vi "PQbinaryTuples.vi"(8 "error in (no error)":errorcluster, 10 "res":u64) -> (0 "error out":errorcluster, 1 "PQbinaryTuples":i64, 2 "res out":u64)   [LabVIEW 2019, in "libpqlv64.lvlib"]
doc: "Returns 1 if the PGresult contains binary data and 0 if it contains text data.\nThis function is deprecated (except for its use in connection with COPY), because it is possible for a single PGresult to contain text data in some columns and binary data in others. PQfformat is preferred. PQbinaryTuples returns 1 only if all columns of the result are binary (format 1)."
uses:
  libpqlv64.lvlib
  libpq.dll
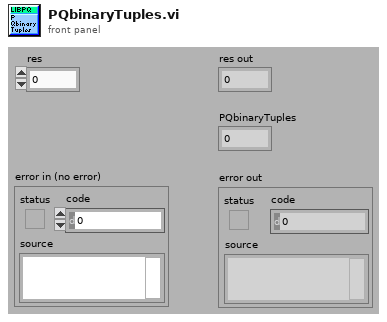
[diagram p1: front panel]
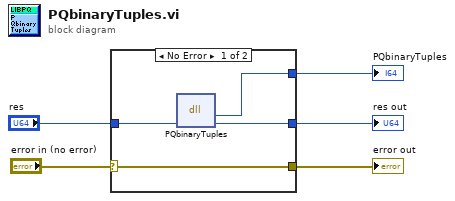
[diagram p0: block diagram]
diagram:
  n1 = case shown="No Error" "error in (no error)" {
    selector: "error in (no error)" -> [w9 w11]
    tunnel: [w9 w11] -> w4
    tunnel: [w8 _] -> w3
    tunnel: "res" -> [w7 w10]
    tunnel: [w6 w10] -> w1
    frame No Error {
      n2 = dll-call lib="libpq.*" fn="PQbinaryTuples"("res"=w7) -> ("PQbinaryTuples"=w8:i64, "res"=w6:u64)  [unwired: 3 in, 2 out]
    }
    frame Error {
    }
  }
  "PQbinaryTuples" <- w3
  "error out" <- w4
  "res out" <- w1
